vi "GetHandleByType.vi"(1 "Type":i16) -> (0 "Handle":i32)   [LabVIEW 2012]
uses:
  Madlib.dll
panel:
  # "Acquires a handle to a specific device. Can be\nused as a subVI."
  # "USB 1.1       USB 2.0\nSingle Axis                      4096            8193\nSingle Axis(20 bit)                              8705\nNanoGuage                      8192           \nThree Axis                       4144           8195\nTip / Tilt Z (16 bit)                             8275\nThree Axis (20 bit)        4656           8707\nTip / Tilt Z (20 bit)         4651           8787"
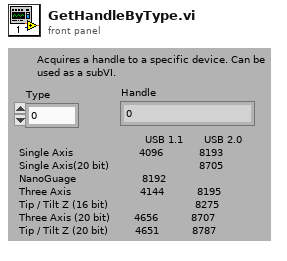
[diagram p1: front panel]
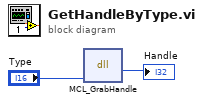
[diagram p0: block diagram]
diagram:
  n1 = dll-call lib="C:/Users/Labview/Desktop/SRR/Madlib_x64/Labview Examples/MADLib.dll" fn="MCL_GrabHandle"("serial"="Type") -> (→"Handle":i32)  [unwired: 4 in, 2 out]
